vi "TrajectoryUtil_WritePathWeaverJSON.vi"(8 "error in (no error)":errorcluster, 10 "inTRAJECTORY":T1 {"States"."POSE"."ROTATION"."SIN" format="%13.4f"; "States"."POSE"."ROTATION"."COS" format="%13.4f"; "States"."POSE"."ROTATION"."VALUE" format="%13.4f"; "States"."POSE"."TRANSLATION"."Y" format="%14.3f"; "States"."POSE"."TRANSLATION"."X" format="%14.3f"; "TotalTImeSecs" format="%20.3f"}, 11 "FileName":string="trajectory.json") -> (0 "error out":errorcluster)   [LabVIEW 2019]
doc: "Imports a Trajectory from a PathWeaver-style JSON file.\n\nParameters:\n - FileName - File name string of the json file to import from\n - Error In - Error cluster (not used)\n\nReturns:\n - Trajectory - Trajectory data structure\n - Error out - Returned error cluster"
uses:
  <vilib>/Rock Robotics/WPI/ThirdParty/JAS_Junk/TrajLib/TRANSLATION2D.ctl
  <vilib>/Rock Robotics/WPI/ThirdParty/JAS_Junk/TrajLib/Trajectory_Library.lvlib
  <vilib>/Rock Robotics/WPI/ThirdParty/JAS_Junk/TrajLib/ROTATION2D.ctl
  <vilib>/Rock Robotics/WPI/ThirdParty/JAS_Junk/TrajLib/POSE2D.ctl
  <vilib>/Rock Robotics/WPI/ThirdParty/JAS_Junk/TrajLib/TRAJ_STATE.ctl
  <vilib>/Rock Robotics/WPI/ThirdParty/JAS_Junk/TrajLib/TRAJECTORY.ctl
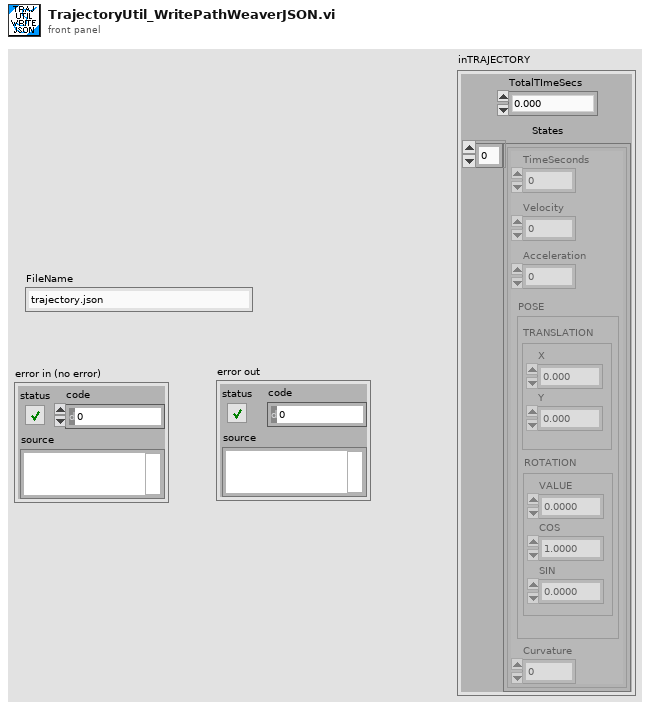
[diagram p1: front panel]
types:
  T1 = typedef "Trajectory_Library.lvlib/TRAJECTORY.ctl" = cluster{"TotalTImeSecs":dbl, "States":T2[]}
  T2 = typedef "Trajectory_Library.lvlib/TRAJ_STATE.ctl" = cluster{"TimeSeconds":dbl, "Velocity":dbl, "Acceleration":dbl, "POSE":T3, "Curvature":dbl}
  T3 = typedef "Trajectory_Library.lvlib/POSE2D.ctl" = cluster{"TRANSLATION":T4, "ROTATION":T5}
  T4 = typedef "Trajectory_Library.lvlib/TRANSLATION2D.ctl" = cluster{"X":dbl, "Y":dbl}
  T5 = typedef "Trajectory_Library.lvlib/ROTATION2D.ctl" = cluster{"VALUE":dbl, "COS":dbl, "SIN":dbl}
  T6 = enum16{"open", "replace", "create", "open or create", "replace or create", "replace or create with confirmation"}
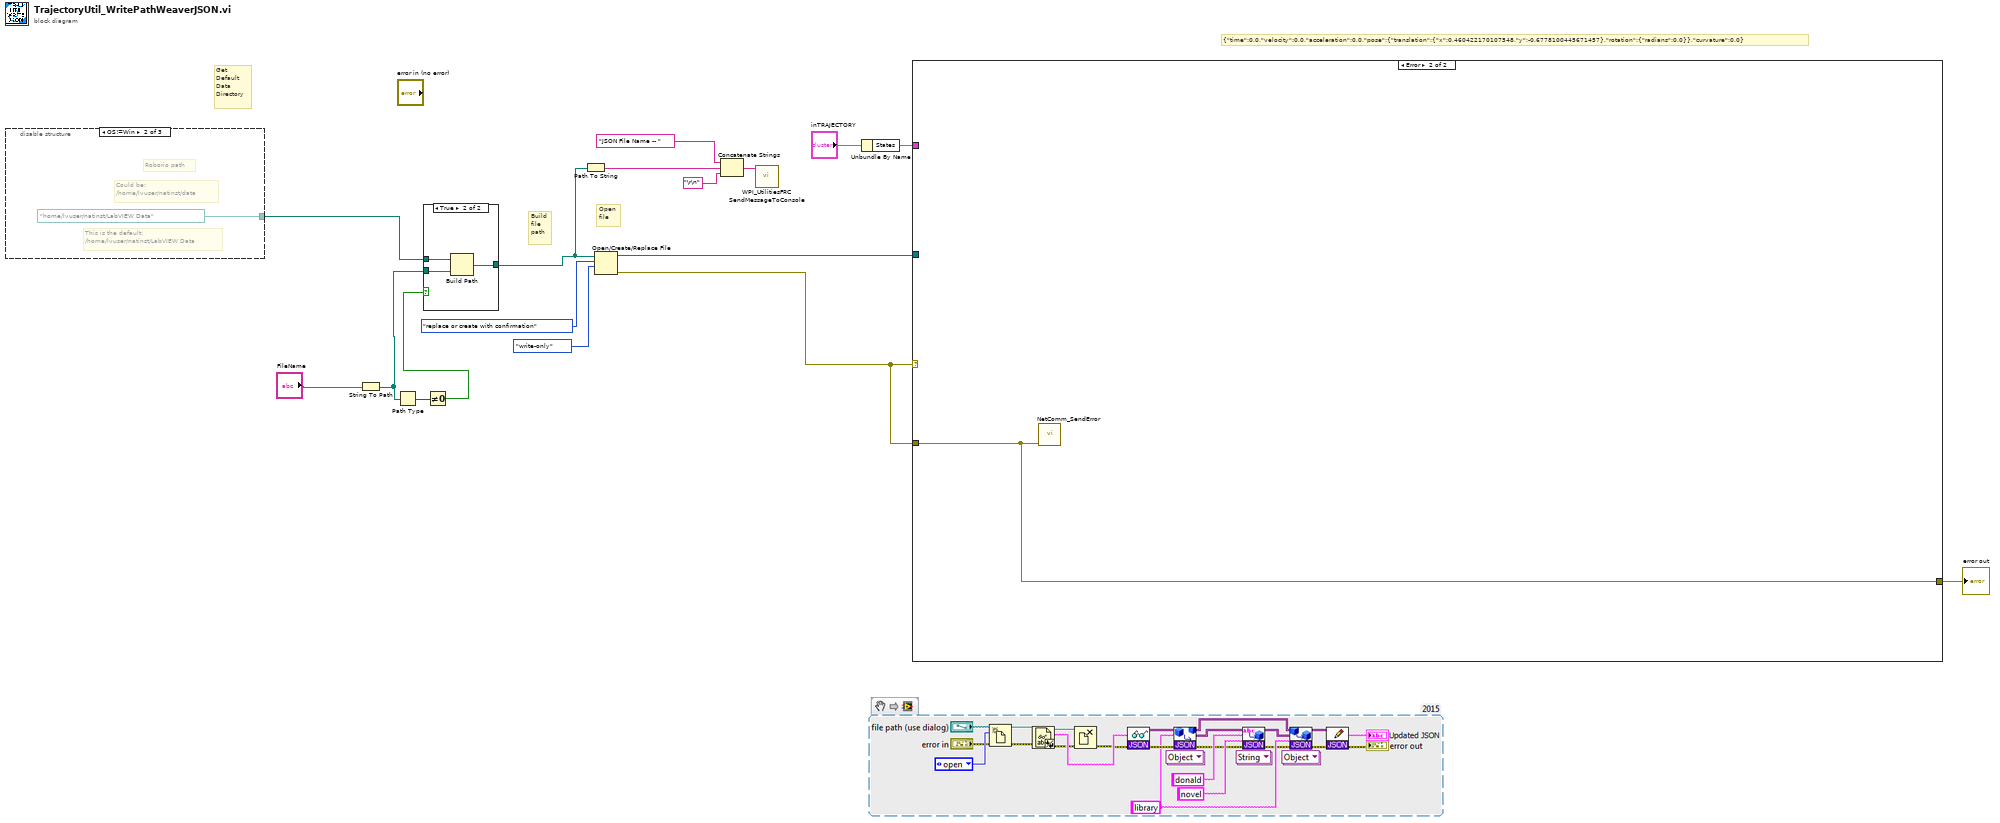
[diagram p0: block diagram]
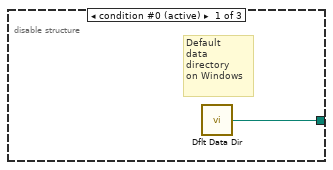
[diagram p3: hidden frame]
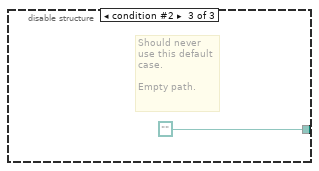
[diagram p4: hidden frame]
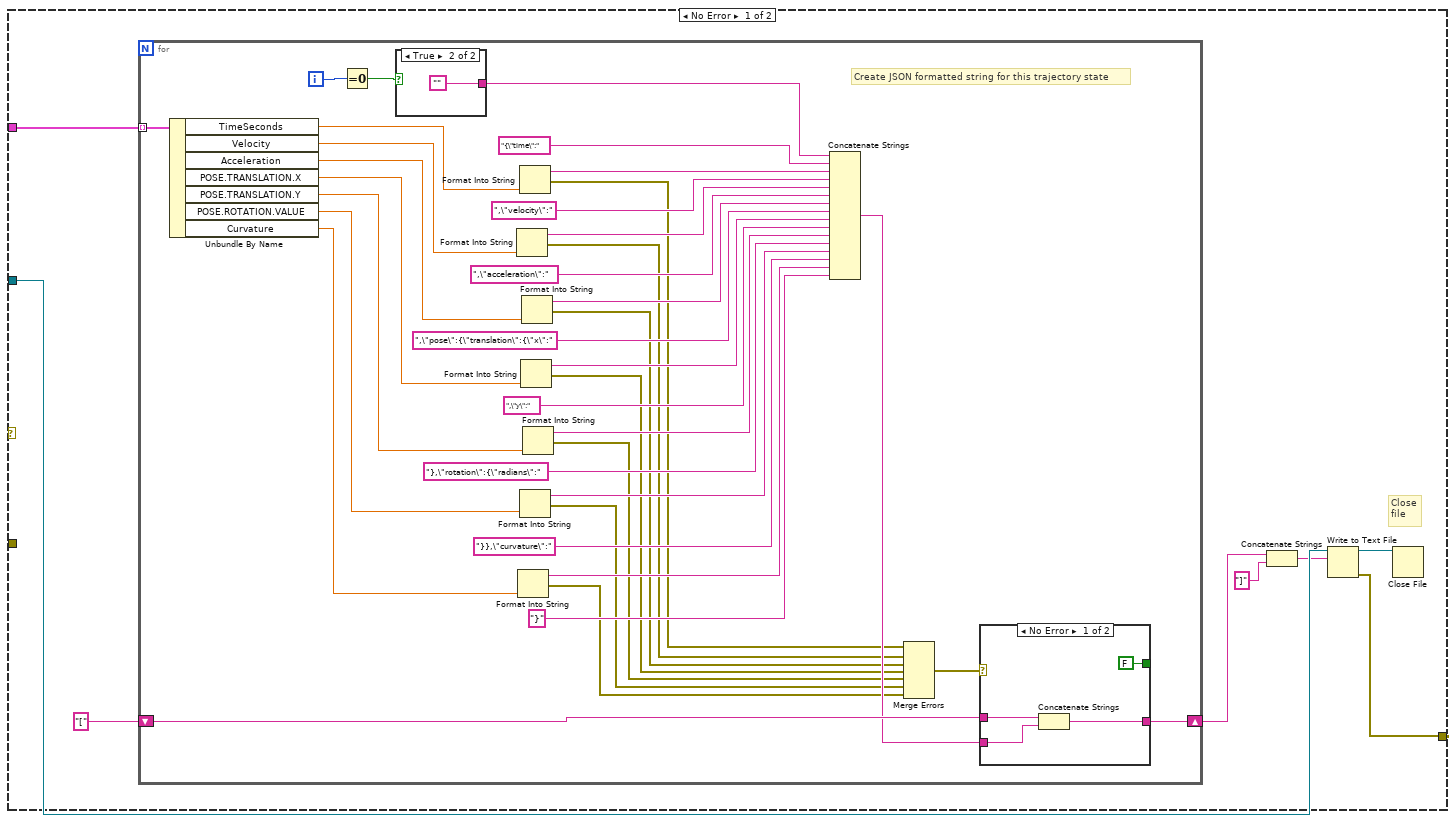
[diagram p5: hidden frame]
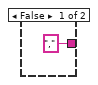
[diagram p6: hidden frame]
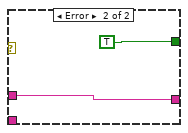
[diagram p7: hidden frame]
diagram:
  # "{\"time\":0.0,\"velocity\":0.0,\"acceleration\":0.0,\"pose\":{\"translation\":{\"x\":0.460422170107548,\"y\":-0.6778100445671457},\"rotation\":{\"radians\":0.0}},\"curvature\":0.0}"
  # "Get\nDefault\nData\nDirectory"
  # "Open\nfile"
  # "Build\nfile\npath"
  n1 = disable-structure shown="OS!=Win" {
    disable-tunnel: [w18 path "/home/lvuser/natinst/LabVIEW Data" path ""] -> w9
    frame condition #0 (active) {
      # "Default\ndata\ndirectory\non Windows"
      n2 = call <vilib>:"Dflt Data Dir.vi"() -> ("App:Default Data Directory"=w18:path)
    }
    frame condition #1 {
      # "This is the default:\n/home/lvuser/natinst/LabVIEW Data"
      # "Could be:\n/home/lvuser/natinst/data"
      # "Roborio path"
    }
    frame condition #2 {
      # "Should never\nuse this default\ncase.\n\nEmpty path."
    }
  }
  n3 = String To Path(string="FileName") -> (path=w6:path)
  n4 = Path Type(1:w6) -> (0:w5:i16)
  n5 = Not Equal To 0?(x=w5) -> (x != 0?=w4:bool)
  n6 = case shown="True" w4 {
    tunnel: [w21 w24] -> w15
    tunnel: w9 -> [_ w23]
    tunnel: w6 -> [w21 w22]
    frame False {
    }
    frame True {
      n7 = Build Path(base path=w23, name or relative path=w22) -> (appended path=w24:path)
    }
  }
  n8 = Path To String(path=w15) -> (string=w13:string)
  n9 = Open/Create/Replace File(file path (use dialog)=w15, operation (0:open)=T6."replace or create with confirmation", access (0:read/write)=enum16{"read/write", "read-only", "write-only"}."write-only") -> (refnum out=w1:refnum<file>, error out=w10:errorcluster)  [unwired: 3 in, 1 out]
  n10 = Concatenate Strings("JSON File Name -- ", w13, "\r\n") -> (w11:string)
  n11 = call <vilib>:"WPI_UtilitiesFRC SendMessageToConsole.vi"("Message"=w11) -> ()  [unwired: 14 in, 1 out]
  n12 = Unbundle By Name("inTRAJECTORY") -> ("States"=w2:T2[])
  n13 = case shown="Error" w10 {
    tunnel: w10 -> [_ w78]
    tunnel: [w26 w78] -> w8
    tunnel: w2 -> [w32 _]
    tunnel: w1 -> [w28 _]
    frame No Error {
      # "Close\nfile"
      n14 = for {
        tunnel: w32 -> [w68] mode=indexing
        shift-right: [w41] -> w30
        shift-left: "[" -> [w42]
        i -> [w67]
        # "Create JSON formatted string for this trajectory state"
        n15 = Unbundle By Name(w68) -> ("TimeSeconds"=w49:dbl, "Velocity"=w48:dbl, "Acceleration"=w47:dbl, "POSE.TRANSLATION.X"=w46:dbl, "POSE.TRANSLATION.Y"=w45:dbl, "POSE.ROTATION.VALUE"=w44:dbl, "Curvature"=w43:dbl)
        n16 = Equal To 0?(x=w67) -> (x = 0?=w66:bool)
        n17 = case shown="True" w66 {
          tunnel: ["," ""] -> w65
          frame False {
          }
          frame True {
          }
        }
        n18 = Format Into String(w48) -> (resulting string=w61:string, error out=w38:errorcluster)  [unwired: 3 in]
        n19 = Format Into String(w43) -> (resulting string=w51:string, error out=w33:errorcluster)  [unwired: 3 in]
        n20 = Format Into String(w49) -> (resulting string=w63:string, error out=w39:errorcluster)  [unwired: 3 in]
        n21 = Format Into String(w44) -> (resulting string=w53:string, error out=w34:errorcluster)  [unwired: 3 in]
        n22 = Format Into String(w46) -> (resulting string=w57:string, error out=w36:errorcluster)  [unwired: 3 in]
        n23 = Format Into String(w47) -> (resulting string=w59:string, error out=w37:errorcluster)  [unwired: 3 in]
        n24 = Format Into String(w45) -> (resulting string=w55:string, error out=w35:errorcluster)  [unwired: 3 in]
        n25 = Concatenate Strings(w65, "{\"time\":", w63, ",\"velocity\":", w61, ",\"acceleration\":", w59, ",\"pose\":{\"translation\":{\"x\":", w57, ",\"y\":", w55, "},\"rotation\":{\"radians\":", w53, "}},\"curvature\":", w51, "}") -> (w40:string)
        n26 = Merge Errors(w39, w38, w37, w36, w35, w34, w33) -> (w69:errorcluster)
        n27 = case shown="No Error" w69 {
          tunnel: [FALSE TRUE] -> _
          tunnel: w42 -> [w74 w76]
          tunnel: [w73 w76] -> w41
          tunnel: w40 -> [w72 _]
          frame No Error {
            n28 = Concatenate Strings(w74, w72) -> (w73:string)
          }
          frame Error {
          }
        }
      }
      n29 = Concatenate Strings(w30, "]" ("string")) -> (w27:string)
      n30 = Write to Text File(file (use dialog)=w28, text=w27) -> (refnum out=w25:refnum<file>, error out=w26:errorcluster)  [unwired: 2 in, 1 out]
      n31 = Close File(refnum=w25) -> ()  [unwired: 1 in, 2 out]
    }
    frame Error {
      n32 = call <vilib>:"NetComm_SendError.vi"("error in (no error)"=w78) -> ()  [unwired: 11 in]
    }
  }
  "error out" <- w8
